vi "Global.vi"() -> ()   [LabVIEW 2016]
panel:
  in  "Chat":string
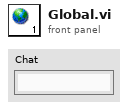
[diagram p1: front panel]
diagram:
